vi "Is Bookmark.vi"(7 "Bookmark":T1, 8 "Error In":errorcluster, 11 "VI Bookmark":T2) -> (0 "Error Out":errorcluster, 3 "Is Bookmark":bool)   [LabVIEW 2017, in "Bookmark Manager.lvlib"]
uses:
  Bookmark Manager.lvlib
  Controls/VI Bookmark.ctl
  Controls/VI Information.ctl
  Controls/Application Information.ctl
  Toolkit/Typedefs/Bookmark Tags.ctl
  Toolkit/Toolkit.lvlib
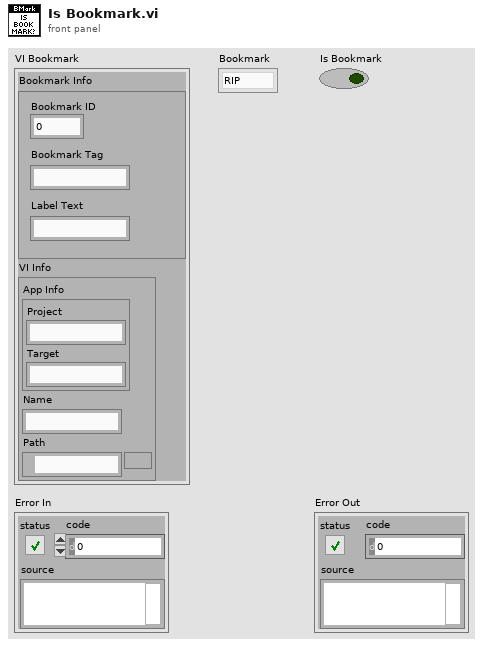
[diagram p1: front panel]
types:
  T1 = typedef "Toolkit.lvlib/Bookmark Tags.ctl" = enum16{"RIP", "Zombie"}
  T2 = typedef "Bookmark Manager.lvlib/VI Bookmark.ctl" = cluster{"Bookmark Info":cluster{"Bookmark ID":u32, "Bookmark Tag":string, "Label Text":string}, "VI Info":T3}
  T3 = typedef "Bookmark Manager.lvlib/VI Information.ctl" = cluster{"App Info":T4, "Name":string, "Path":path}
  T4 = typedef "Bookmark Manager.lvlib/Application Information.ctl" = cluster{"Project":string, "Target":string}
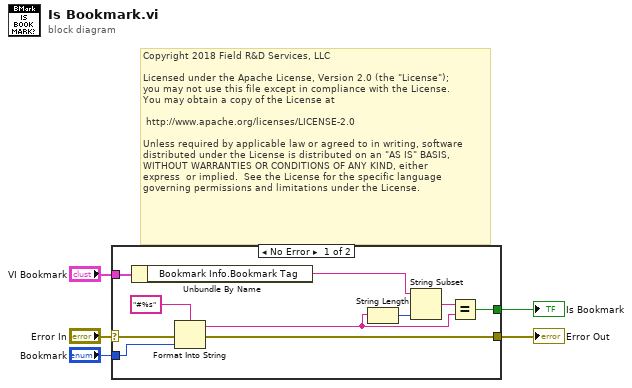
[diagram p0: block diagram]
diagram:
  # "Copyright 2018 Field R&D Services, LLC\n\nLicensed under the Apache License, Version 2.0 (the \"License\");\nyou may not use this file except in compliance with the License.\nYou may obtain a copy of the License at\n\n\thttp://www.apache.org/licenses/LICENSE-2.0\n\nUnless required by applicable law or agreed to in writing, software\ndistributed under the License is distributed on an \"AS IS\" BASIS,\nWITHOUT WARRANTIES OR CONDITIONS OF ANY KIND, either \nexpress  or implied.  See the License for the specific language \ngoverning permissions and limitations under the License."
  n1 = case shown="No Error" "Error In" {
    selector: "Error In" -> [w6 w16]
    tunnel: "VI Bookmark" -> [w14 _]
    tunnel: [w12 _] -> w4
    tunnel: "Bookmark" -> [w10 _]
    tunnel: [w7 w16] -> w2
    frame No Error {
      n2 = Unbundle By Name(w14) -> ("Bookmark Info.Bookmark Tag"=w13:string)
      n3 = Format Into String(format string="#%s", error in=w6, w10) -> (resulting string=w8:string, error out=w7:errorcluster)  [unwired: 1 in]
      n4 = String Length(string=w8) -> (length=w15:i32)
      n5 = String Subset(string=w13, length (rest)=w15) -> (substring=w11:string)  [unwired: 1 in]
      n6 = Equal?(x=w11, y=w8) -> (x = y?=w12:bool)
    }
    frame Error {
    }
  }
  "Is Bookmark" <- w4
  "Error Out" <- w2
